vi "Script Error VI.vi"(4 "Error Code":i32, 5 "Module type":T1, 6 "Error Name":string, 7 "Error Arguments Window Ref":refnum<vi>, 8 "error in":errorcluster, 10 "Library Path":path, 11 "VI Ref Error in":refnum<vi>) -> (0 "error out":errorcluster)   [LabVIEW 2019, in "Panther Dashboard.lvlib"]
uses:
  Panther Dashboard.lvlib
  Module type--enum.ctl
  <vilib>/Utility/traverseref.llb/TRef TravTarget.ctl
  <vilib>/Utility/miscctls.llb/LVPositionTypeDef.ctl
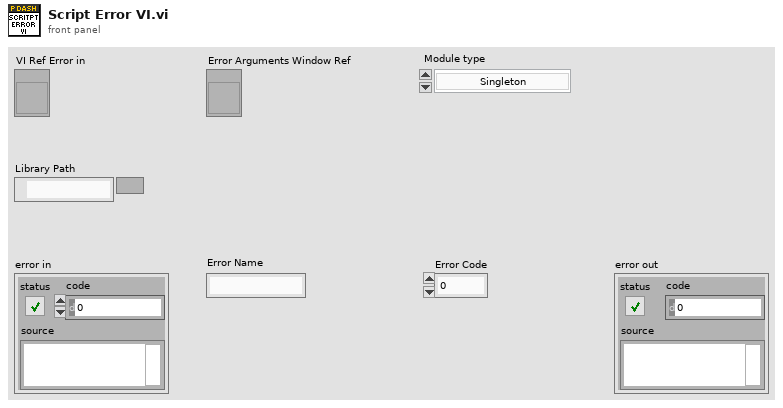
[diagram p1: front panel]
types:
  T1 = typedef "Panther Dashboard.lvlib/Module type--enum.ctl" = enum16{"Singleton", "Cloneable"}
  T2 = typedef "TRef TravTarget.ctl" = enum16{"FP", "BD", "Other"}
  T3 = typedef "LVPositionTypeDef.ctl" = cluster{"Left":i32, "Top":i32}
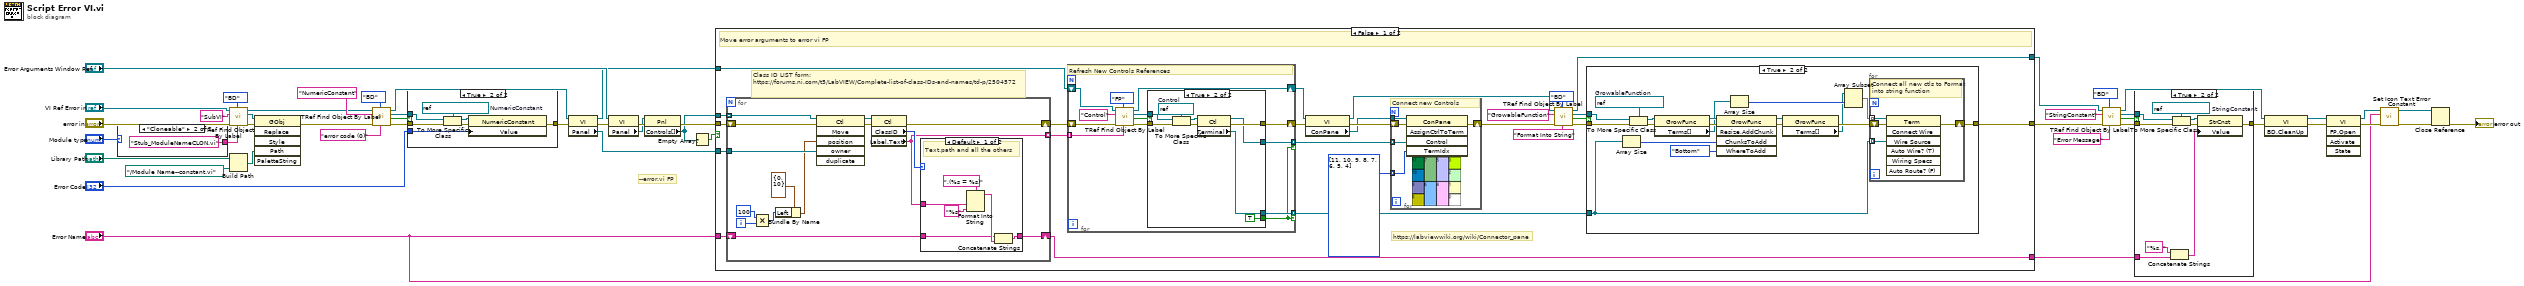
[diagram p0: block diagram]
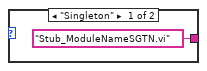
[diagram p2: hidden frame]
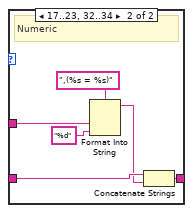
[diagram p5: hidden frame]
diagram:
  # "--error.vi FP"
  n1 = case shown="\"Cloneable\"" "Module type" {
    tunnel: ["Stub_ModuleNameSGTN.vi" ("Label") "Stub_ModuleNameCLON.vi" ("Label")] -> w29
    frame "Singleton" {
    }
    frame "Cloneable" {
    }
  }
  n2 = call <vilib>:"TRef Find Object By Label.vi"("Label"=w29, "Traverse Target"=TRef_TravTarget."BD", "error in (no error)"="error in", "Class Name"="SubVI", "VI Ref"="VI Ref Error in") -> ("error out"=w50:errorcluster, "Found Obj Ref"=w30:refnum<vi>, "dup VI Ref"=w25:refnum<vi>)  [unwired: 3 in, 1 out]
  n3 = Build Path(base path="Library Path", name or relative path=path "../Module Name--constant.vi") -> (appended path=w33:path)
  n4 = invoke class="GObj" method="Replace"(reference=w30, error in=w50, "Path"=w33) -> (error out=w48:errorcluster)  [unwired: 3 in, 5 out]
  n5 = call <vilib>:"TRef Find Object By Label.vi"("Label"="error code (0)", "Traverse Target"=TRef_TravTarget."BD", "error in (no error)"=w48, "Class Name"="NumericConstant", "VI Ref"=w25) -> ("error out"=w47:errorcluster, "Found?"=w24:bool, "Found Obj Ref"=w23:refnum<vi>, "dup VI Ref"=w12:refnum<vi>)  [unwired: 3 in]
  n6 = case shown="True" w24 {
    tunnel: w47 -> [w53 w60]
    tunnel: w23 -> [_ w57]
    tunnel: "Error Code" -> [_ w54]
    tunnel: [w53 w58] -> w42
    frame False {
    }
    frame True {
      w56 = refnum<vi> refnum  # NumericConstant
      n7 = To More Specific Class(target class=w56, reference=w57, error in=w60) -> (specific class reference=w55:refnum<vi>, error out=w59:errorcluster)
      n8 = property class="NumericConstant"(reference=w55, error in=w59, "Value"=w54) -> (error out=w58:errorcluster)  [unwired: 1 out]
    }
  }
  n9 = property class="VI"(reference=w12, error in=w42) -> (reference out=w10:refnum<vi>, error out=w43:errorcluster, "Panel"=w13:refnum<vi>)
  n10 = property class="VI"(reference="Error Arguments Window Ref", error in=w43) -> (error out=w45:errorcluster, "Panel"=w16:refnum<vi>)  [unwired: 1 out]
  n11 = property class="Pnl"(reference=w16, error in=w45) -> (error out=w44:errorcluster, "Controls[]"=w14:refnum<vi>[])  [unwired: 1 out]
  n12 = Empty Array?(array=w14) -> (empty?=w15:bool)
  n13 = case shown="False" w15 {
    tunnel: w44 -> [w85 w166]
    tunnel: w14 -> [w69 _]
    tunnel: w13 -> [w78 _]
    tunnel: [w83 w166] -> w41
    tunnel: "Error Name" -> [w77 w165]
    tunnel: [w76 w165] -> w3
    tunnel: w10 -> [w66 w164]
    tunnel: [w75 w164] -> w9
    frame False {
      # "https://labviewwiki.org/wiki/Connector_pane"
      # "Class ID LIST form:\nhttps://forums.ni.com/t5/LabVIEW/Complete-list-of-class-IDs-and-names/td-p/2504572"
      # "Move error arguments to error vi FP"
      n14 = for {
        tunnel: w69 -> [w143] mode=indexing
        tunnel: w78 -> [w142]
        shift-right: [w144] -> w82
        shift-left: w85 -> [w146]
        shift-right: [w137] -> w76
        shift-left: w77 -> [w138]
        tunnel: [w136] -> w68 mode=indexing
        i -> [w134]
        n15 = Multiply(x=100, y=w134) -> (x*y=w133:i32)
        n16 = Bundle By Name(cluster=T3 {"Left"=0, "Top"=10} ("position"), "Left"=w133) -> (w135:T3)
        n17 = invoke class="Ctl" method="Move"(reference=w143, error in=w146, "position"=w135, "owner"=w142) -> (reference out=w140:refnum<vi>, error out=w145:errorcluster)  [unwired: 2 in, 4 out]
        n18 = property class="Ctl"(reference=w140, error in=w145) -> (error out=w144:errorcluster, "ClassID"=w139:u32, "Label.Text"=w136:string)  [unwired: 1 out]
        n19 = case shown="Default" w139 {
          tunnel: w138 -> [w148 w158]
          tunnel: [w149 w157] -> w137
          tunnel: w136 -> [w147 w156]
          frame Default {
            # "Text,path and all the others"
            n20 = Format Into String(format string=",(%s = %s)", w147, "%s" ("string")) -> (resulting string=w150:string)  [unwired: 2 in, 1 out]
            n21 = Concatenate Strings(w148, w150) -> (w149:string)
          }
          frame 17..23, 32..34 {
            # "Numeric"
            n22 = Format Into String(format string=",(%s = %s)", w156, "%d" ("string")) -> (resulting string=w153:string)  [unwired: 2 in, 1 out]
            n23 = Concatenate Strings(w158, w153) -> (w157:string)
          }
        }
      }
      n24 = for {
        tunnel: w68 -> [w118] mode=indexing
        shift-right: [w119] -> w81
        shift-left: w82 -> [w121]
        tunnel: [w114] -> w67 mode=indexing if=w109
        shift-right: [w111] -> w65
        shift-left: w66 -> [w113]
        tunnel: [w110] -> w62 mode=indexing if=w109
        # "Refresh New Controls References"
        n25 = call <vilib>:"TRef Find Object By Label.vi"("Label"=w118, "Traverse Target"=TRef_TravTarget."FP", "error in (no error)"=w121, "Class Name"="Control", "VI Ref"=w113) -> ("error out"=w120:errorcluster, "Found?"=w112:bool, "Found Obj Ref"=w116:refnum<vi>, "dup VI Ref"=w111:refnum<vi>)  [unwired: 3 in]
        n26 = case shown="True" w112 {
          tunnel: w116 -> [_ w128]
          tunnel: [_ w125] -> w114
          tunnel: w120 -> [w122 w131]
          tunnel: [w122 w129] -> w119
          tunnel: [_ TRUE] -> w109
          tunnel: [_ w123] -> w110
          frame False {
          }
          frame True {
            w126 = refnum<vi> refnum  # Control
            n27 = To More Specific Class(target class=w126, reference=w128, error in=w131) -> (specific class reference=w127:refnum<vi>, error out=w130:errorcluster)
            n28 = property class="Ctl"(reference=w127, error in=w130) -> (reference out=w123:refnum<vi>, error out=w129:errorcluster, "Terminal"=w125:refnum<vi>)
          }
        }
      }
      n29 = property class="VI"(reference=w65, error in=w81) -> (reference out=w64:refnum<vi>, error out=w80:errorcluster, "ConPane"=w63:refnum<vi>)
      n30 = for {
        tunnel: w63 -> [w161]
        shift-right: [w162] -> w79
        shift-left: w80 -> [w163]
        tunnel: w62 -> [w160] mode=indexing
        tunnel: i32[] [11, 10, 9, 8, 7, 6, 5, 4] -> [w159] mode=indexing
        # "Connect new Controls"
        n31 = invoke class="ConPane" method="AssignCtrlToTerm"(reference=w161, error in=w163, "Control"=w160, "TermIdx"=w159) -> (error out=w162:errorcluster)  [unwired: 1 in, 4 out]
      }
      n32 = call <vilib>:"TRef Find Object By Label.vi"("Label"="Format Into String", "Traverse Target"=TRef_TravTarget."BD", "error in (no error)"=w79, "Class Name"="GrowableFunction", "VI Ref"=w64) -> ("error out"=w84:errorcluster, "Found?"=w72:bool, "Found Obj Ref"=w71:refnum<vi>, "dup VI Ref"=w75:refnum<vi>)  [unwired: 3 in]
      n33 = case shown="True" w72 {
        tunnel: w84 -> [w86 w104]
        tunnel: w71 -> [_ w98]
        tunnel: [w86 w99] -> w83
        tunnel: w67 -> [_ w87]
        frame False {
        }
        frame True {
          w97 = refnum<vi> refnum  # GrowableFunction
          n34 = Array Size(array=w87) -> (size(s)=w95:i32)
          n35 = To More Specific Class(target class=w97, reference=w98, error in=w104) -> (specific class reference=w93:refnum<vi>, error out=w103:errorcluster)
          n36 = property class="GrowFunc"(reference=w93, error in=w103) -> (reference out=w92:refnum<vi>, error out=w101:errorcluster, "Terms[]"=w91:refnum<vi>[])
          n37 = invoke class="GrowFunc" method="Resize.AddChunk"(reference=w92, error in=w101, "ChunksToAdd"=w95, "WhereToAdd"=enum8{"Bottom", "Top"}."Bottom" ("Where To Add")) -> (reference out=w94:refnum<vi>, error out=w102:errorcluster)  [unwired: 1 in, 3 out]
          n38 = Array Size(array=w91) -> (size(s)=w90:i32)
          n39 = property class="GrowFunc"(reference=w94, error in=w102) -> (error out=w100:errorcluster, "Terms[]"=w89:refnum<vi>[])  [unwired: 1 out]
          n40 = Array Subset(array=w89, index=w90) -> (w88:refnum<vi>[])  [unwired: 1 in]
          n41 = for {
            tunnel: w88 -> [w106] mode=indexing
            tunnel: w87 -> [w105] mode=indexing
            shift-right: [w107] -> w99
            shift-left: w100 -> [w108]
            # "Connect all new ctls to Format into string function"
            n42 = invoke class="Term" method="Connect Wire"(reference=w106, error in=w108, "Wire Source"=w105) -> (error out=w107:errorcluster)  [unwired: 4 in, 6 out]
          }
        }
      }
    }
    frame True {
      # "No Error Arguments"
    }
  }
  n43 = call <vilib>:"TRef Find Object By Label.vi"("Label"="Error Message", "Traverse Target"=TRef_TravTarget."BD", "error in (no error)"=w41, "Class Name"="StringConstant", "VI Ref"=w9) -> ("error out"=w46:errorcluster, "Found?"=w19:bool, "Found Obj Ref"=w18:refnum<vi>, "dup VI Ref"=w11:refnum<vi>)  [unwired: 3 in]
  n44 = case shown="True" w19 {
    tunnel: w46 -> [w167 w176]
    tunnel: w18 -> [_ w173]
    tunnel: [w167 w174] -> w40
    tunnel: w3 -> [_ w170]
    frame False {
    }
    frame True {
      w172 = refnum<vi> refnum  # StringConstant
      n45 = Concatenate Strings("%s, " ("string"), w170) -> (w169:string)
      n46 = To More Specific Class(target class=w172, reference=w173, error in=w176) -> (specific class reference=w171:refnum<vi>, error out=w175:errorcluster)
      n47 = property class="StrCnst"(reference=w171, error in=w175, "Value"=w169) -> (error out=w174:errorcluster)  [unwired: 1 out]
    }
  }
  n48 = invoke class="VI" method="BD.CleanUp"(reference=w11, error in=w40) -> (reference out=w5:refnum<vi>, error out=w39:errorcluster)  [unwired: 1 in, 1 out]
  n49 = invoke class="VI" method="FP.Open"(reference=w5, error in=w39) -> (reference out=w4:refnum<vi>, error out=w38:errorcluster)  [unwired: 3 in, 3 out]
  n50 = call "Set Icon Text Error Constant.vi"("error in"=w38, "Text"="Error Name", "VI in"=w4) -> ("error out"=w37:errorcluster, "VI out"=w1:refnum<vi>)  [unwired: 7 in]
  n51 = Close Reference(reference=w1, error in (no error)=w37) -> (error out=→"error out":errorcluster)
